vi "Acquire.vi"(8 "error in (no error)":errorcluster, 11 "Diode IV in":refnum<class "Diode IV.lvclass">) -> (0 "error out":errorcluster, 3 "Diode IV out":refnum<class "Diode IV.lvclass">)   [LabVIEW 2015, in "Diode Characterization.lvlib" / "Diode IV.lvclass"]
uses:
  Diode IV.lvclass
  <userlib>/Common Components/Hardware/DMM/DMM.lvclass
  <userlib>/Common Components/Hardware/PSU/PSU.lvclass
  <vilib>/ActorFramework/Actor/Actor.lvclass/Actor.ctl
  <vilib>/ActorFramework/Message Enqueuer/Message Enqueuer.lvclass/Message Enqueuer.ctl
  <vilib>/ActorFramework/Message Enqueuer/Init from Existing Queue.vi
  <vilib>/ActorFramework/Message Enqueuer/Enqueue.vi
  <vilib>/ActorFramework/Message Priority Queue/Priority Enqueue.vi
  <vilib>/ActorFramework/Message Enqueuer/Message Enqueuer.lvclass
  <userlib>/Common Components/Measurement Actor/Messages/Measure Msg/Measure Msg.lvclass
  <userlib>/Common Components/Measurement Actor/Measurement.lvclass
  <vilib>/ActorFramework/Actor/Actor.lvclass
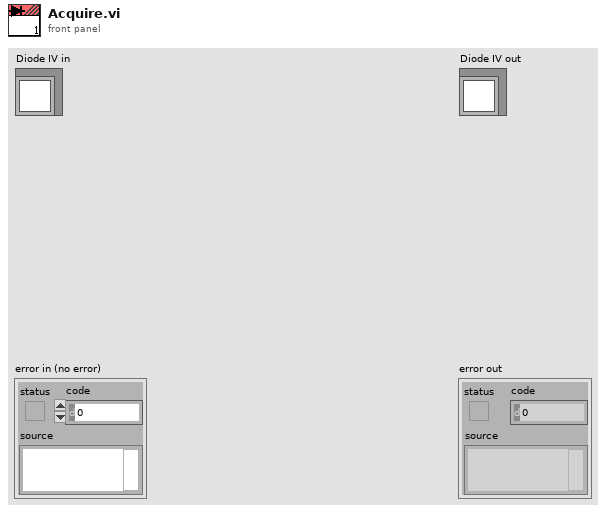
[diagram p1: front panel]
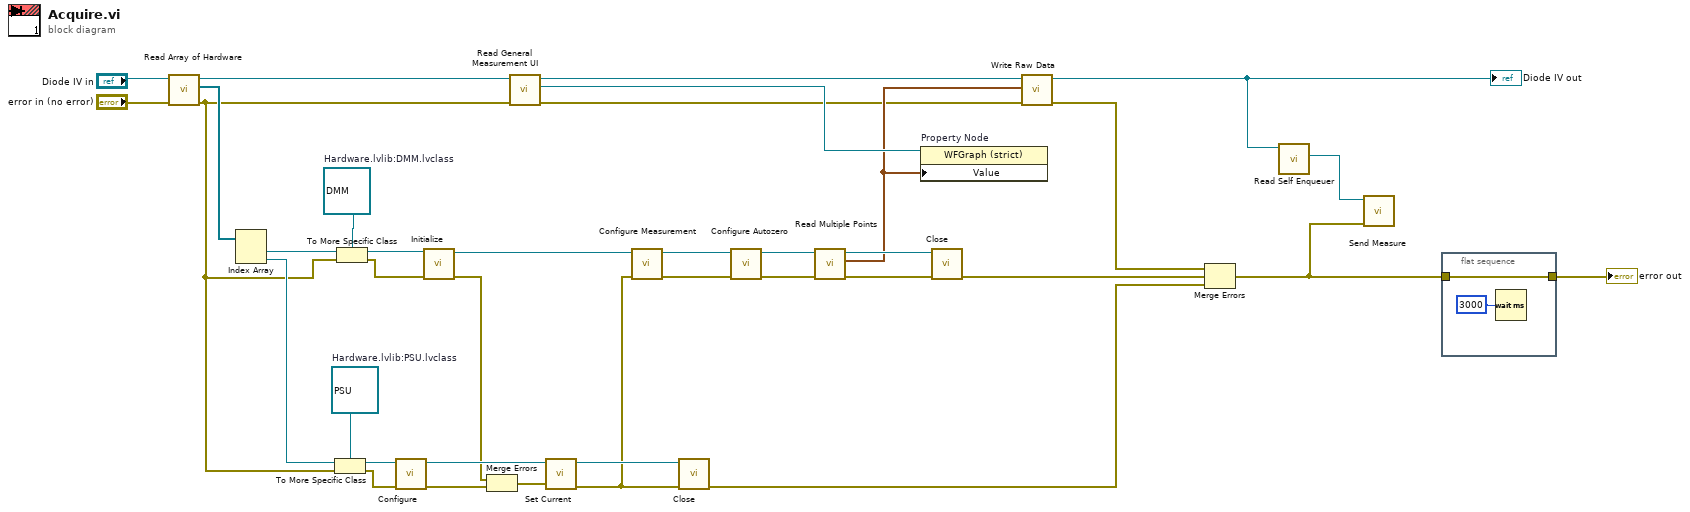
[diagram p0: block diagram]
diagram:
  w5 = refnum<class "PSU.lvclass"> refnum  # Hardware.lvlib:PSU.lvclass
  w6 = refnum<class "DMM.lvclass"> refnum  # Hardware.lvlib:DMM.lvclass
  n1 = call <userlib>:"Read Array of Hardware.vi"("error in (no error)"="error in (no error)", "Measurement in"="Diode IV in") -> ("error out"=w7:errorcluster, "Array of Hardware"=w26:refnum<class "Hardware.lvclass">[], "Measurement out"=w4:refnum<class "Diode IV.lvclass">)  [unwired: 7 in]
  n2 = Index Array(array=w26) -> (element #1=w27:refnum<class "Hardware.lvclass">, element #2=w28:refnum<class "Hardware.lvclass">)  [unwired: 2 in]
  n3 = To More Specific Class(target class=w5, reference=w28, error in=w7) -> (specific class reference=w35:refnum<class "PSU.lvclass">, error out=w1:errorcluster)
  n4 = To More Specific Class(target class=w6, reference=w27, error in=w7) -> (specific class reference=w33:refnum<class "DMM.lvclass">, error out=w2:errorcluster)
  n5 = call-dynamic "Configure.vi"("error in (no error)"=w1, "PSU in"=w35) -> ("error out"=w12:errorcluster, "PSU out"=w36:refnum<class "PSU.lvclass">)  [unwired: 8 in]
  n6 = call-dynamic "Initialize.vi"("error in (no error)"=w2, "Analog in"=w33) -> ("error out"=w11:errorcluster, "Analog out"=w32:refnum<class "DMM.lvclass">)  [unwired: 8 in]
  n7 = Merge Errors(w11, w12) -> (w13:errorcluster)
  n8 = call <userlib>:"Read General Measurement UI.vi"("error in (no error)"=w7, "Measurement in"=w4) -> ("error out"=w14:errorcluster, "General Measurement UI"=w23:refnum<vi>, "Measurement out"=w21:refnum<class "Diode IV.lvclass">)  [unwired: 7 in]
  n9 = call-dynamic "Set Current.vi"("error in (no error)"=w13, "PSU in"=w36) -> ("error out"=w15:errorcluster, "PSU out"=w37:refnum<class "PSU.lvclass">)  [unwired: 8 in]
  n10 = call-dynamic "Configure Measurement.vi"("error in (no error)"=w15, "DMM in"=w32) -> ("error out"=w16:errorcluster, "DMM out"=w31:refnum<class "DMM.lvclass">)  [unwired: 8 in]
  n11 = call-dynamic "Close.vi"("error in (no error)"=w15, "PSU in"=w37) -> ("error out"=w10:errorcluster)  [unwired: 8 in, 1 out]
  n12 = call-dynamic "Configure Autozero.vi"("error in (no error)"=w16, "DMM in"=w31) -> ("error out"=w34:errorcluster, "DMM out"=w30:refnum<class "DMM.lvclass">)  [unwired: 8 in]
  n13 = call-dynamic "Read Multiple Points.vi"("error in (no error)"=w34, "DMM in"=w30) -> ("error out"=w17:errorcluster, "Waveform"=w22:waveform(dbl), "DMM out"=w29:refnum<class "DMM.lvclass">)  [unwired: 7 in]
  n14 = property on="Property Node" class="WFGraph (strict)"(reference=w23, "Value"=w22) -> ()  [unwired: 1 in, 2 out]
  n15 = call-dynamic "Close.vi"("error in (no error)"=w17, "DMM in"=w29) -> ("error out"=w9:errorcluster)  [unwired: 8 in, 1 out]
  n16 = call "Write Raw Data.vi"("error in (no error)"=w14, "Raw Data"=w22, "Diode I-V in"=w21) -> ("error out"=w8:errorcluster, "Diode I-V out"=w19:refnum<class "Diode IV.lvclass">)  [unwired: 7 in]
  "Diode IV out" <- w19
  n17 = Merge Errors(w8, w9, w10) -> (w3:errorcluster)
  n18 = call <vilib>:"Read Self Enqueuer.vi"("Actor"=w19) -> ("Self Enqueuer"=w18:refnum<class "Message Enqueuer.lvclass">)  [unwired: 10 in]
  n19 = call <userlib>:"Send Measure.vi"("error in (no error)"=w3, "Message Enqueuer in"=w18) -> ()  [unwired: 8 in, 2 out]
  n20 = flat-sequence {
    tunnel: w3 -> [w38]
    tunnel: [w38] -> w20
    frame #0 {
      n21 = Wait (ms)(milliseconds to wait=u32 3000) -> ()  [unwired: 1 out]
    }
  }
  "error out" <- w20
